vi "31 Intro to Audio.vi"() -> ()   [LabVIEW 2019]
uses:
  _Subs/OpenDiagram/Open_XControl.xctl
  <vilib>/measure/NI_MABase.lvlib
panel:
  in  "offset":dbl format="%0.2p"
  in  "sampling info":cluster{"Fs":dbl, "#s":dbl}={"Fs"=1000.0, "#s"=1000.0} {"Fs" format="%.2p"}
  in  "signal type":T1(ring)
  in  "phase":dbl format="%.2p"
  in  "amplitude":dbl=1.0 format="%0.2p"
  in  "frequency":dbl=10.0 format="%0.2p"
  out "Waveform Graph":waveform(dbl)(graph)
  in  "stop":bool
  in  "OpenDiag":refnum<vi>(xcontrol)
  # "31 Intro to Audio\nThis code demonstrates how to graph and play a generated wave signal.  \n\nInstructions:\n1. Hit run and play around with the generated wave on the graph."
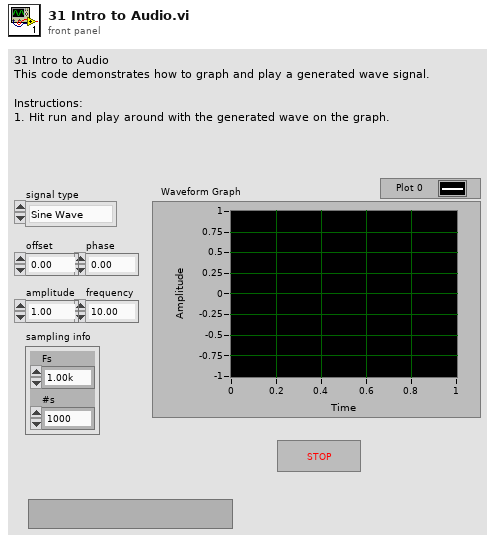
[diagram p1: front panel]
types:
  T1 = enum16{"Sine Wave", "Triangle Wave", "Square Wave", "Sawtooth Wave"}
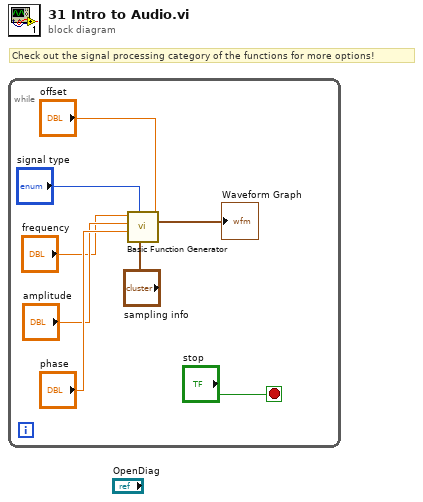
[diagram p0: block diagram]
diagram:
  # "Check out the signal processing category of the functions for more options!"
  n1 = while {
    stop <- "stop" stop-if-true
    n2 = call <vilib>:"Basic Function Generator.vi"("offset"="offset", "sampling info"="sampling info", "signal type"="signal type", "phase"="phase", "amplitude"="amplitude", "frequency"="frequency") -> ("signal out"=→"Waveform Graph":waveform(dbl))  [unwired: 3 in, 2 out]
  }
